vi "VoltageRatioInputSetSensorType.vi"(0 "error in (no error)":errorcluster, 2 "Sesnor Type":u32(ring) caption="Sensor Type" items=["SENSOR_TYPE_VOLTAGERATIO"=0, "SENSOR_TYPE_1101_SHARP_2D120X"=11011, "SENSOR_TYPE_1101_SHARP_2Y0A21"=11012, "SENSOR_TYPE_1101_SHARP_2Y0A02"=11013, "SENSOR_TYPE_1102"=11020, "SENSOR_TYPE_1103"=11030, "SENSOR_TYPE_1104"=11040, "SENSOR_TYPE_1105"=11050, "SENSOR_TYPE_1106"=11060, "SENSOR_TYPE_1107"=11070, "SENSOR_TYPE_1108"=11080, "SENSOR_TYPE_1109"=11090, "SENSOR_TYPE_1110"=11100, "SENSOR_TYPE_1111"=11110, "SENSOR_TYPE_1112"=11120, "SENSOR_TYPE_1113"=11130, "SENSOR_TYPE_1115"=11150, "SENSOR_TYPE_1116"=11160, "SENSOR_TYPE_1118_AC"=11181, "SENSOR_TYPE_1118_DC"=11182, "SENSOR_TYPE_1119_AC"=11191, "SENSOR_TYPE_1119_DC"=11192, "SENSOR_TYPE_1120"=11200, "SENSOR_TYPE_1121"=11210, "SENSOR_TYPE_1122_AC"=11221, "SENSOR_TYPE_1122_DC"=11222, "SENSOR_TYPE_1124"=11240, "SENSOR_TYPE_1125_HUMIDITY"=11251, "SENSOR_TYPE_1125_TEMPERATURE"=11252, "SENSOR_TYPE_1126"=11260, "SENSOR_TYPE_1128"=11280, "SENSOR_TYPE_1129"=11290, "SENSOR_TYPE_1131"=11310, "SENSOR_TYPE_1134"=11340, "SENSOR_TYPE_1136"=11360, "SENSOR_TYPE_1137"=11370, "SENSOR_TYPE_1138"=11380, "SENSOR_TYPE_1139"=11390, "SENSOR_TYPE_1140"=11400, "SENSOR_TYPE_1141"=11410, "SENSOR_TYPE_1146"=11460, "SENSOR_TYPE_3120"=31200, "SENSOR_TYPE_3121"=31210, "SENSOR_TYPE_3122"=31220, "SENSOR_TYPE_3123"=31230, "SENSOR_TYPE_3130"=31300, "SENSOR_TYPE_3520"=35200, "SENSOR_TYPE_3521"=35210, "SENSOR_TYPE_3522"=35220], 3 "Device In":u64) -> (7 "error out":errorcluster, 10 "Device Out":u64)   [LabVIEW 2020, in "Phidget Voltage Ratio Input.lvlib"]
doc: "${SensorType:Header}"
uses:
  <instrlib>/Phidgets/Phidget Voltage Ratio Input/Phidget Voltage Ratio Input.lvlib
  <instrlib>/Phidgets/Phidget Common/Phidget Common.lvlib
  phidget22.dll
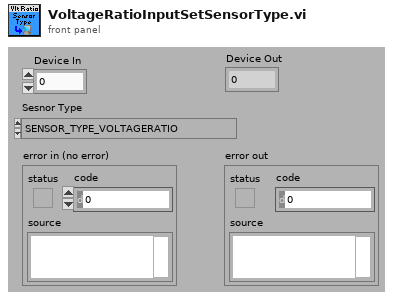
[diagram p1: front panel]
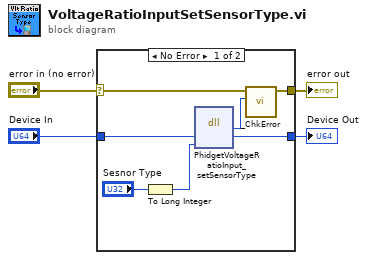
[diagram p0: block diagram]
diagram:
  n1 = case shown="No Error" "error in (no error)" {
    selector: "error in (no error)" -> [w9 w13]
    tunnel: [w8 w13] -> w3
    tunnel: "Device In" -> [w11 w12]
    tunnel: [w10 w12] -> w1
    frame No Error {
      n2 = To Long Integer(number="Sesnor Type") -> (32bit integer=w5:i32)
      n3 = dll-call lib="phidget22.*" fn="PhidgetVoltageRatioInput_setSensorType"("phid"=w11, "interval"=w5) -> ("return type"=w7:i32, "phid"=w10:u64)  [unwired: 4 in, 2 out]
      n4 = call <instrlib>:"_ChkError.vi"("Return Code"=w7, "error in (no error)"=w9) -> ("error out"=w8:errorcluster)  [unwired: 9 in]
    }
    frame Error {
    }
  }
  "error out" <- w3
  "Device Out" <- w1
